vi "Add History.vi"(7 "Data IN":T2={"Impulse Positions"=[], "Old Impulse positions for Undo"=[], "No. Imp"=0, "Parameter Time Series"=[], "Parameter Impuls Series"=[], "Experiment Parameters"={"Freq"=0.0, "Vel"=0, "Acc"=0, "Stimulus"=""}, "Autosort File"=refnum, "Data File"={"Data Channels"=[], "Sample Rate"=0, "Channel List"=[]}, "Experiment data path"=path "/Macintosh HD/Users/patrick/Studium/Diploma Thesis/Data Analysis", "Image data path"=path "/Macintosh HD/Users/patrick/Studium/Diploma Thesis/Data Analysis", "LVS data path"=path "/Macintosh HD/Users/patrick/Studium/Diploma Thesis/Data Analysis", "Raw copy path"=path "/Macintosh HD/Users/patrick/Studium/Diploma Thesis/Data Analysis", "filename"="No file selected", "desaccading parameters"={"Tolerance"=0, "Acc Range"=0.0, "Sample Rate"=0, "Impulse Plane 2"=enum."Other", "Impulse dir"=FALSE}, "Experiment Parameters 2"={"Subject"="", "Strain"="", "Rotation plane"="", "Experimenter"="", "Trial"=0.0, "Time"=0.0}, "Excel"={"Excel._Application"=refnum, "Use Excel"=FALSE, "Worksheet SINE"=refnum, "Row SINE"=0, "Worksheet TRANS"=refnum, "Row TRANS"=0}, "Session Config File"=refnum, "Autosort Parameter Set"=1, "EMA Version"="", "desacc "={"Threshold 1 [Acc]"=1617.080808080808, "Threshold 2 [% of TH1]"=67, "tolerance"=5, "Search WD "=0.19090909090909092, " always use TH2"=TRUE, "Range"=3.2323232323232323, "Max time"=200.0, "Min time"=20.0, "Velocity Threshold"=67}, "Cycle Nr for Saccades"={"POS"=0, "NEG"=0}, "Undo Counter"=0, "History Length"=0, "Redo Counter"=0, "Histpry Position"=0, "Raw Data File"={"Data Channels"=[], "Sample Rate"=0, "Channel List"=[]}, "calibration name"="No file selected"} {"Parameter Time Series"."time offset" format="%.3f"; "Parameter Time Series"."Gain" format="%.1f"; "Parameter Time Series"."Offset" format="%.1f"; "Parameter Time Series"."List 1" items=["Motor-Pos", "Motor-Vel", "Lx Position-in-Head", "Ly Position-in-Head", "Lz Position-in-Head", "Lx Velocity-in-Head", "Ly Velocity-in-Head", "Lz Velocity-in-Head", "Ll Velocity-in-Head", "Lr Velocity-in-Head", "Lx Accel-in-Head", "Ly Accel-in-Head", "Lz Accel-in-Head", "Rx Position-in-Head", "Ry Position-in-Head", "Rz Position-in-Head", "Rx Velocity-in-Head", "Ry Velocity-in-Head", "Rz Velocity-in-Head", "Rl Velocity-in-Head", "Rr Velocity-in-Head", "Rx Accel-in-Head", "Ry Accel-in-Head", "Rz Accel-in-Head", "Global Trigger", "", "", ""]; "Parameter Impuls Series"."Gain" format="%.1f"; "Parameter Impuls Series"."Offset" format="%.1f"}, 10 "Impulse Positions":T1(array[cluster]) {"Amplitude offset" format="%.2f"}) -> (5 "Data OUT":T2={"Impulse Positions"=[], "Old Impulse positions for Undo"=[], "No. Imp"=0, "Parameter Time Series"=[], "Parameter Impuls Series"=[], "Experiment Parameters"={"Freq"=0.0, "Vel"=0, "Acc"=0, "Stimulus"=""}, "Autosort File"=refnum, "Data File"={"Data Channels"=[], "Sample Rate"=0, "Channel List"=[]}, "Experiment data path"=path "/Macintosh HD/Users/patrick/Studium/Diploma Thesis/Data Analysis", "Image data path"=path "/Macintosh HD/Users/patrick/Studium/Diploma Thesis/Data Analysis", "LVS data path"=path "/Macintosh HD/Users/patrick/Studium/Diploma Thesis/Data Analysis", "Raw copy path"=path "/Macintosh HD/Users/patrick/Studium/Diploma Thesis/Data Analysis", "filename"="No file selected", "desaccading parameters"={"Tolerance"=0, "Acc Range"=0.0, "Sample Rate"=0, "Impulse Plane 2"=enum."Other", "Impulse dir"=FALSE}, "Experiment Parameters 2"={"Subject"="", "Strain"="", "Rotation plane"="", "Experimenter"="", "Trial"=0.0, "Time"=0.0}, "Excel"={"Excel._Application"=refnum, "Use Excel"=FALSE, "Worksheet SINE"=refnum, "Row SINE"=0, "Worksheet TRANS"=refnum, "Row TRANS"=0}, "Session Config File"=refnum, "Autosort Parameter Set"=1, "EMA Version"="", "desacc "={"Threshold 1 [Acc]"=1617.080808080808, "Threshold 2 [% of TH1]"=67, "tolerance"=5, "Search WD "=0.19090909090909092, " always use TH2"=TRUE, "Range"=3.2323232323232323, "Max time"=200.0, "Min time"=20.0, "Velocity Threshold"=67}, "Cycle Nr for Saccades"={"POS"=0, "NEG"=0}, "Undo Counter"=0, "History Length"=0, "Redo Counter"=0, "Histpry Position"=0, "Raw Data File"={"Data Channels"=[], "Sample Rate"=0, "Channel List"=[]}, "calibration name"="No file selected"} {"Parameter Time Series"."time offset" format="%.3f"; "Parameter Time Series"."Gain" format="%.1f"; "Parameter Time Series"."Offset" format="%.1f"; "Parameter Time Series"."List 1" items=["Motor-Pos", "Motor-Vel", "Lx Position-in-Head", "Ly Position-in-Head", "Lz Position-in-Head", "Lx Velocity-in-Head", "Ly Velocity-in-Head", "Lz Velocity-in-Head", "Ll Velocity-in-Head", "Lr Velocity-in-Head", "Lx Accel-in-Head", "Ly Accel-in-Head", "Lz Accel-in-Head", "Rx Position-in-Head", "Ry Position-in-Head", "Rz Position-in-Head", "Rx Velocity-in-Head", "Ry Velocity-in-Head", "Rz Velocity-in-Head", "Rl Velocity-in-Head", "Rr Velocity-in-Head", "Rx Accel-in-Head", "Ry Accel-in-Head", "Rz Accel-in-Head", "Global Trigger", "", "", ""]; "Parameter Impuls Series"."Gain" format="%.1f"; "Parameter Impuls Series"."Offset" format="%.1f"})   [LabVIEW 2016]
uses:
  type-defs/TD_Statemachine-Data.ctl
  type-defs/TD_Time Series.ctl
  type-defs/TD_Impulse Parameter.ctl
  core.lvlib
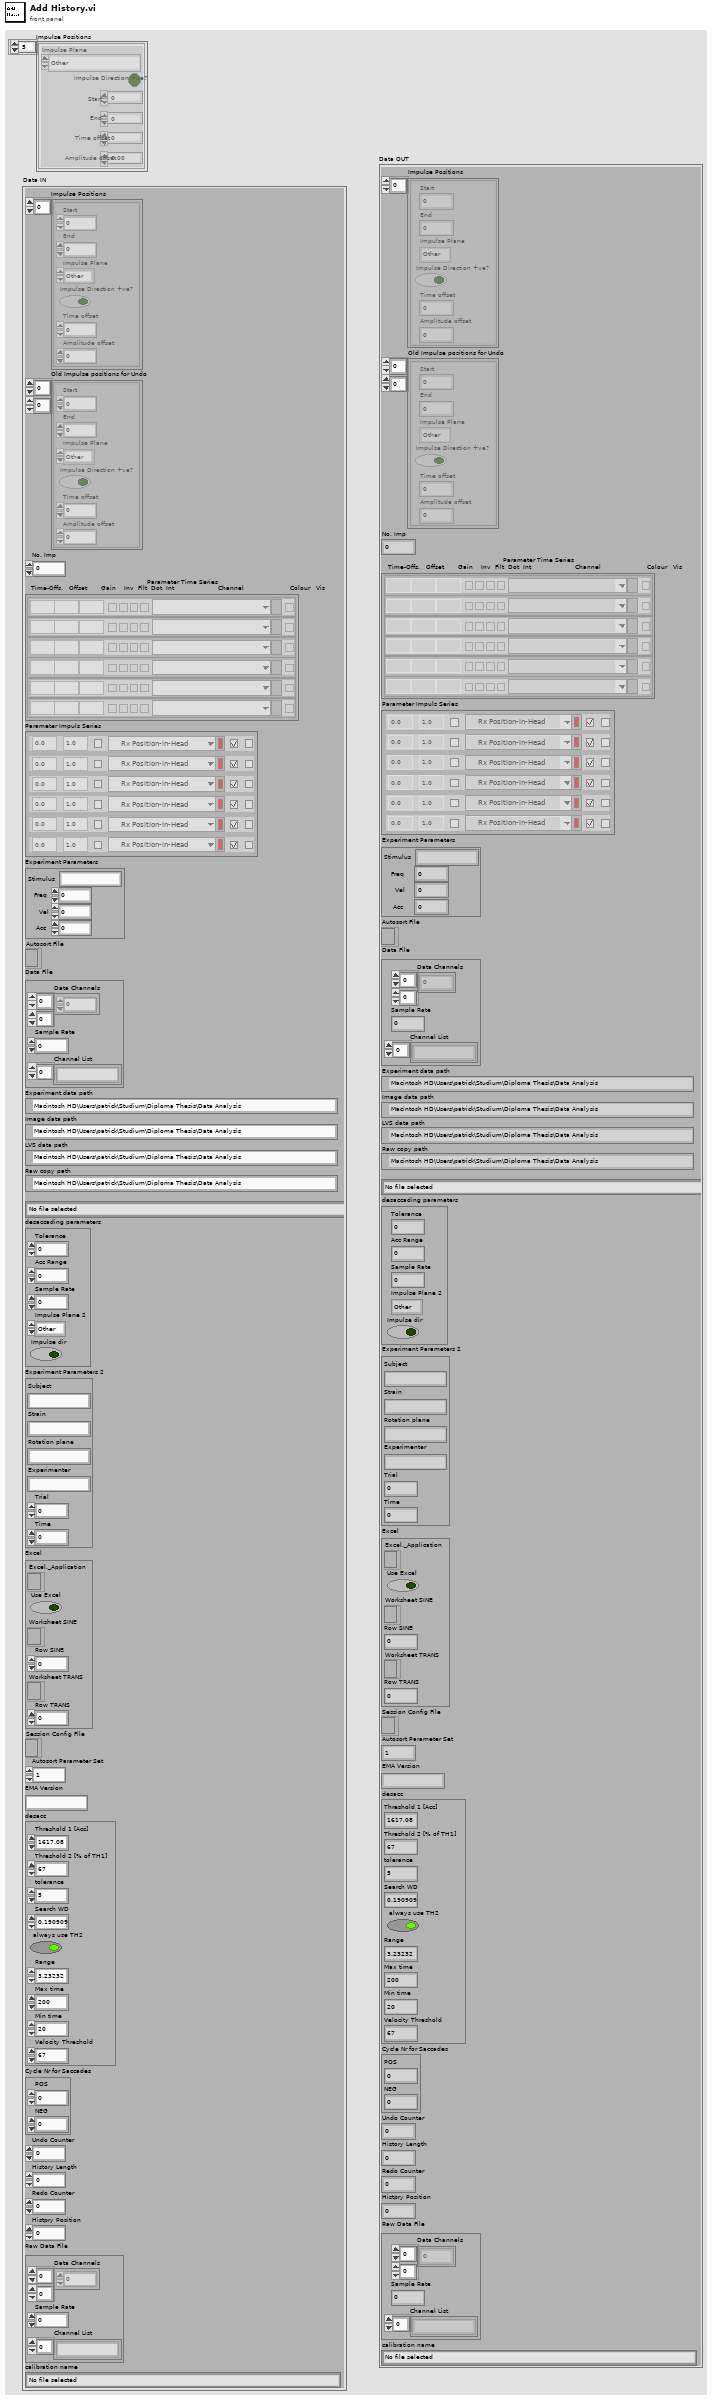
[diagram p1: front panel]
types:
  T1 = cluster{"Start":i32, "End":i32, "Impulse Plane":enum16{"Other", "Yaw", "Pitch", "Roll", "LARP", "RALP"}, "Impulse Direction +ve?":bool, "Time offset":i32, "Amplitude offset":dbl}[]
  T2 = typedef "core.lvlib/TD_Statemachine-Data.ctl" = cluster{"Impulse Positions":cluster{"Start":i32, "End":i32, "Impulse Plane":enum16{"Other", "Yaw", "Pitch", "Roll", "LARP", "RALP"}, "Impulse Direction +ve?":bool, "Time offset":i32, "Amplitude offset":dbl}[], "Old Impulse positions for Undo":cluster{"Start":i32, "End":i32, "Impulse Plane":enum16{"Other", "Yaw", "Pitch", "Roll", "LARP", "RALP"}, "Impulse Direction +ve?":bool, "Time offset":i32, "Amplitude offset":dbl}[][], "No. Imp":i32, "Parameter Time Series":T3, "Parameter Impuls Series":T4, "Experiment Parameters":cluster{"Freq":dbl, "Vel":i32, "Acc":i32, "Stimulus":string}, "Autosort File":refnum<file>, "Data File":cluster{"Data Channels":dbl[][], "Sample Rate":i32, "Channel List":string[]}, "Experiment data path":path, "Image data path":path, "LVS data path":path, "Raw copy path":path, "filename":string, "desaccading parameters":cluster{"Tolerance":i32, "Acc Range":dbl, "Sample Rate":i32, "Impulse Plane 2":enum16{"Other", "Yaw", "Pitch", "Roll", "LARP", "RALP"}, "Impulse dir":bool}, "Experiment Parameters 2":cluster{"Subject":string, "Strain":string, "Rotation plane":string, "Experimenter":string, "Trial":dbl, "Time":dbl}, "Excel":cluster{"Excel._Application":refnum<k7>, "Use Excel":bool, "Worksheet SINE":refnum<k7>, "Row SINE":i32, "Worksheet TRANS":refnum<k7>, "Row TRANS":i32}, "Session Config File":refnum<file>, "Autosort Parameter Set":i32, "EMA Version":string, "desacc ":cluster{"Threshold 1 [Acc]":dbl, "Threshold 2 [% of TH1]":i32, "tolerance":i32, "Search WD ":dbl, " always use TH2":bool, "Range":dbl, "Max time":dbl, "Min time":dbl, "Velocity Threshold":i32}, "Cycle Nr for Saccades":cluster{"POS":i32, "NEG":i32}, "Undo Counter":i32, "History Length":i32, "Redo Counter":i32, "Histpry Position":i32, "Raw Data File":cluster{"Data Channels":dbl[][], "Sample Rate":i32, "Channel List":string[]}, "calibration name":string}
  T3 = typedef "core.lvlib/TD_Time Series.ctl" = cluster{"time offset":dbl, "Offset":dbl, "Gain":dbl, "inverse":bool, "filter data":bool, "dots":bool, "interpolate":bool, "List 1":u16, "Color Box":u32, "Boolean":bool}[]
  T4 = typedef "core.lvlib/TD_Impulse Parameter.ctl" = cluster{"Color":u32, "Visible":bool, "Channel":u16, "Invert":bool, "Desaccade":bool, "Offset":dbl, "Gain":dbl}[]
  T5 = cluster{"Start":i32, "End":i32, "Impulse Plane":enum16{"Other", "Yaw", "Pitch", "Roll", "LARP", "RALP"}, "Impulse Direction +ve?":bool, "Time offset":i32, "Amplitude offset":dbl}[][]
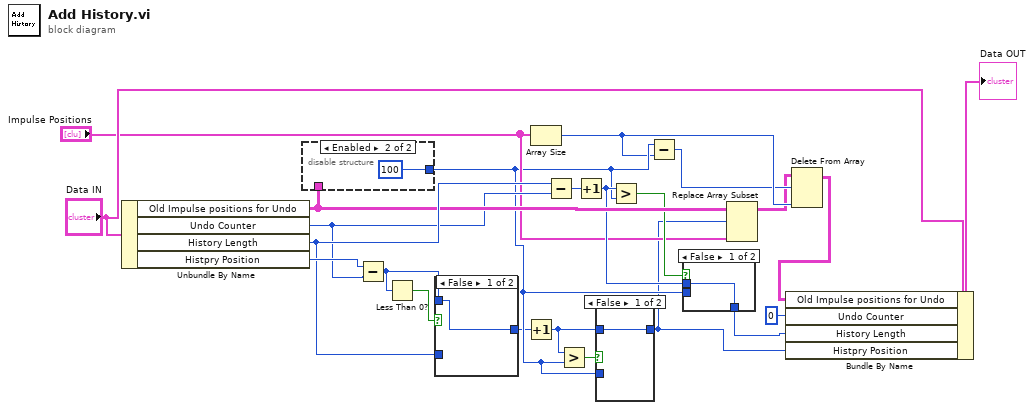
[diagram p0: block diagram]
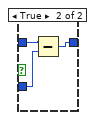
[diagram p2: hidden frame]
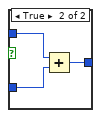
[diagram p4: hidden frame]
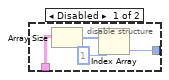
[diagram p5: hidden frame]
diagram:
  n1 = Unbundle By Name("Data IN") -> ("Old Impulse positions for Undo"=w19:T5, "Undo Counter"=w10:i32, "History Length"=w22:i32, "Histpry Position"=w23:i32)
  n2 = disable-structure shown="Enabled" {
    disable-tunnel: w19 -> [w27 _]
    disable-tunnel: [w24 100] -> w8
    frame Disabled {
      n3 = Array Size(array=w27) -> (size(s)=w26:i32[])
      n4 = Index Array(array=w26, index=1) -> (element=w24:i32)
    }
    frame Enabled {
    }
  }
  n5 = Subtract(x=w23, y=w10) -> (x-y=w17:i32)
  n6 = Less Than 0?(x=w17) -> (x < 0?=w18:bool)
  n7 = case shown="False" w18 {
    tunnel: w17 -> [w29 w32]
    tunnel: w22 -> [_ w31]
    tunnel: [w29 w30] -> w2
    frame False {
    }
    frame True {
      n8 = Add(x=w32, y=w31) -> (x+y=w30:i32)
    }
  }
  n9 = Increment(x=w2) -> (x+1=w3:i32)
  n10 = Array Size(array="Impulse Positions") -> (size(s)=w7:i32)
  n11 = Subtract(x=w22, y=w10) -> (x-y=w15:i32)
  n12 = Greater?(x=w3, y=w8) -> (0:w11:bool)
  n13 = Increment(x=w15) -> (x+1=w12:i32)
  n14 = case shown="False" w11 {
    tunnel: w3 -> [w33 w36]
    tunnel: w8 -> [_ w35]
    tunnel: [w33 w34] -> w1
    frame False {
    }
    frame True {
      n15 = Subtract(x=w36, y=w35) -> (x-y=w34:i32)
    }
  }
  n16 = Greater?(x=w12, y=w8) -> (0:w14:bool)
  n17 = Subtract(x=w8, y=w7) -> (x-y=w6:i32)
  n18 = case shown="False" w14 {
    tunnel: w8 -> [_ w38]
    tunnel: [w37 w38] -> w13
    tunnel: w12 -> [w37 _]
    frame False {
    }
    frame True {
    }
  }
  n19 = Replace Array Subset(array=w19, new element="Impulse Positions", index (row)=w1) -> (w5:T5)  [unwired: 1 in]
  n20 = Delete From Array(array=w5, length=w6, index (col)=w7) -> (array with subset deleted=w4:T5)  [unwired: 1 in, 1 out]
  n21 = Bundle By Name(cluster="Data IN", "Old Impulse positions for Undo"=w4, "Undo Counter"=0, "History Length"=w13, "Histpry Position"=w1) -> (→"Data OUT":T2)
